vi "logValues.vi"(0 "Numeric 3":dbl, 1 "Numeric 2":dbl, 2 "Numeric":dbl, 3 "appended path":path) -> ()   [LabVIEW 2018]
panel:
  out "String":string
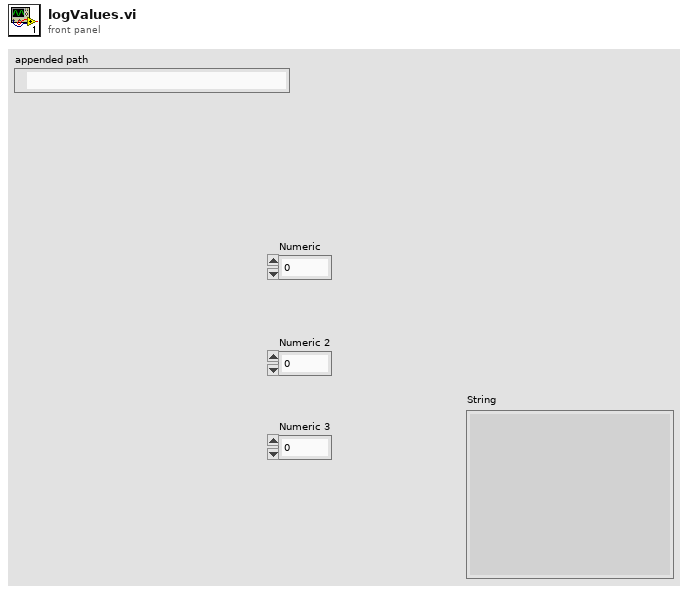
[diagram p1: front panel]
types:
  T1 = enum16{"open", "replace", "create", "open or create", "replace or create", "replace or create with confirmation"}
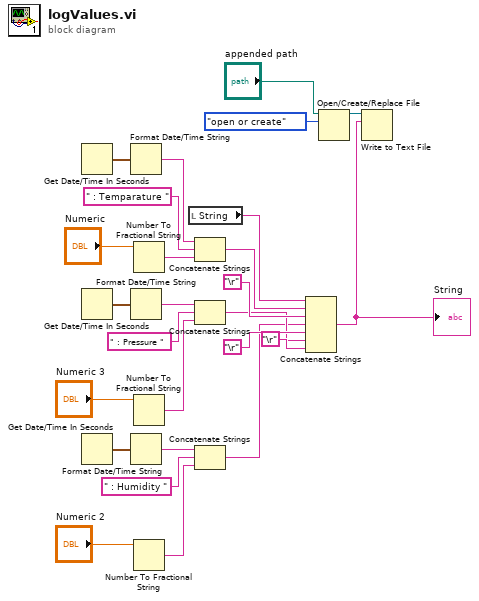
[diagram p0: block diagram]
diagram:
  n1 = Get Date/Time In Seconds() -> (seconds since 1Jan1904=w15:timestamp)
  n2 = Get Date/Time In Seconds() -> (seconds since 1Jan1904=w8:timestamp)
  n3 = Get Date/Time In Seconds() -> (seconds since 1Jan1904=w7:timestamp)
  n4 = Format Date/Time String(seconds (now)=w15) -> (date/time string=w14:string)  [unwired: 2 in]
  n5 = Format Date/Time String(seconds (now)=w8) -> (date/time string=w13:string)  [unwired: 2 in]
  n6 = Format Date/Time String(seconds (now)=w7) -> (date/time string=w6:string)  [unwired: 2 in]
  n7 = Number To Fractional String(number="Numeric") -> (F-format string=w11:string)  [unwired: 3 in]
  n8 = Number To Fractional String(number="Numeric 3") -> (F-format string=w3:string)  [unwired: 3 in]
  n9 = Number To Fractional String(number="Numeric 2") -> (F-format string=w4:string)  [unwired: 3 in]
  n10 = local read "String"() -> (w16:string)
  n11 = Concatenate Strings(w14, " : Temparature ", w11) -> (w10:string)
  n12 = Concatenate Strings(w13, " : Pressure ", w3) -> (w2:string)
  n13 = Concatenate Strings(w6, " : Humidity ", w4) -> (w1:string)
  n14 = Concatenate Strings(w16, w10, "\r", w1, "\r", w2, "\r") -> (w20:string)
  "String" <- w20
  n15 = Open/Create/Replace File(file path (use dialog)="appended path", operation (0:open)=T1."open or create") -> (refnum out=w17:refnum<file>)  [unwired: 4 in, 2 out]
  n16 = Write to Text File(file (use dialog)=w17, text=w20) -> ()  [unwired: 2 in, 3 out]
